vi "Dashboard Main.vi"() -> ()   [LabVIEW 2019]
uses:
  <vilib>/Utility/miscctls.llb/LVRowAndColumnTypeDef.ctl
  <vilib>/event_ctls.llb/eventvkey.ctl
  <vilib>/MakerHub/LINX/Public/Peripherals/Analog/Analog Read 1 Chan.vi
  <vilib>/MakerHub/LINX/Public/Peripherals/Analog/Analog Read N Chans.vi
  <vilib>/MakerHub/LINX/Private/Local IO/LinxAnalogRead.vi
  <vilib>/MakerHub/LINX/Public/Utilities/Check Channel.vi
  <vilib>/Rock Robotics/Network Tables/NT Read Numeric Array.vi
  <vilib>/Rock Robotics/WPI/Dashboard/WPI_DashboardLogging Global.vi
  <vilib>/MakerHub/LINX/Public/Utilities/Open Serial.vi
  <vilib>/MakerHub/LINX/Private/Utilties/Generate Error.vi
  <vilib>/MakerHub/LINX/LMH-LINX.lvlib
panel:
  in  "Camera Settings Right":T1={"Frame Rate"=30, "Compression"=30, "Size"=1, "DB Camera Config"=FALSE} {"Frame Rate" scale=1.0..30.0; "Compression" scale=100.0..-1.0; "Size" items=["640x480", "320x240", "160x120"]}
  in  "Camera Name Right":string(combo)="No Camera Selection"
  out "Camera Perf":string
  in  "Camera Settings":T1={"Frame Rate"=30, "Compression"=30, "Size"=1, "DB Camera Config"=FALSE} {"Frame Rate" scale=1.0..30.0; "Compression" scale=100.0..-1.0; "Size" items=["640x480", "320x240", "160x120"]}
  in  "TCP":refnum<k5>
  in  "Rec Mode":enum32{"Stop", "Record", "Playback"}(radio)
  out "Robot IP":string
  out "Image Message":string="Timeout in Camera Communications"
  in  "Dashboard Tab":T2(tab)
  in  "Select Auto":string(combo)="Select Autonomous ..."
  out "NT Connection":bool
  out "MotorChart R":cluster{"Numeric":dbl, "Numeric":dbl}(graph)
  out "MotorChart L":cluster{"Numeric":dbl, "Numeric":dbl}(graph)
  out "MotorSliders R":cluster{"MotorSlide1":dbl, "MotorSlide2":dbl} {"MotorSlide2" scale=-1.0..1.0 scale format="%#_2e"; "MotorSlide1" scale=-1.0..1.0 scale format="%#_2e"}
  out "MotorSliders L":cluster{"MotorSlide1":dbl, "MotorSlide2":dbl} {"MotorSlide2" scale=-1.0..1.0 scale format="%#_2e"; "MotorSlide1" scale=-1.0..1.0 scale format="%#_2e"}
  out "Gyro":dbl(knob) scale=0.0..360.0
  out "JS1 Z":dbl(slide) scale=-1.0..1.0 scale format="%#_2e"
  out "JS1 Graph":cluster{"X":dbl, "Y":dbl}[](graph)
  out "JS1 Buttons":T3
  out "JS2 Z":dbl(slide) scale=-1.0..1.0 scale format="%#_2e"
  out "JS2 Graph":cluster{"X":dbl, "Y":dbl}[](graph)
  out "JS2 Buttons":T3
  out "Mode":T4(ring)=enum."Auto Disabled"
  out "Right Camera Perf":cluster{"Bandwidth (Mbps)":dbl, "FPS":dbl}
  out "Voltage":dbl(slide) scale=0.0..5.0
  out "Camera Image Right":T5(plugin-control)
  in  "DB/String 9":string
  in  "DB/String 8":string
  in  "DB/String 7":string
  in  "DB/String 6":string
  in  "DB/String 5":string
  in  "DB/String 4":string
  in  "DB/String 3":string
  in  "DB/String 2":string
  in  "DB/String 1":string
  in  "DB/String 0":string
  in  "DB/Slider 0":dbl(slide) scale=0.0..5.0
  in  "DB/Slider 1":dbl(slide) scale=0.0..5.0
  in  "DB/Slider 2":dbl(slide) scale=0.0..5.0
  in  "DB/Slider 3":dbl(slide) scale=0.0..5.0
  out "DB/LED 3":bool
  out "DB/LED 2":bool
  out "DB/LED 1":bool
  out "DB/LED 0":bool
  in  "DB/Button 3":bool
  in  "DB/Button 2":bool
  in  "DB/Button 1":bool
  in  "DB/Button 0":bool caption="New Name"
  in  "Test Slider":dbl(slide) scale=0.0..100.0 scale format="%#_3g"
  in  "On/Off":bool caption="Solenoid"
  in  "Test Name":u16(ring) items=["Select the test to run..."]
  in  "Test Tree":string(tree)
  in  "Motor":cluster{"Value":dbl, "Enable":bool} {"Value" scale=-1.0..1.0 scale format="%#_3g"}
  out "Progress":T6 {"Test Progress" scale=0.0..100.0}
  in  "Rev/Fwd":cluster{"Forward":bool, "Reverse":bool}
  in  "Test Ring":u16(ring) items=["Monochrome", "Color"]
  out "Cmd Status":string
  in  "Execute Command":bool
  in  "Command Params":string[][](table)
  in  "Command Selection":i32(listbox)
  in  "CheckList":i32(listbox)
  out "Tree":string(tree)
  out "Camera Image":T5(plugin-control)
  out "Background":bool
  in  "Camera Name":string(combo)="No Camera Selection"
  # "HW"
  # "HW"
  # "Joysticks"
  # "Drive Motors"
  # "Front"
  # "Right"
  # "Left"
  # "Back"
  # "This tab is a great place for autonomous settings and robot-specific values.\nPlace controls and indicators inside this tab and match name to\nDashboard Variables on robot. You can also delete this comment."
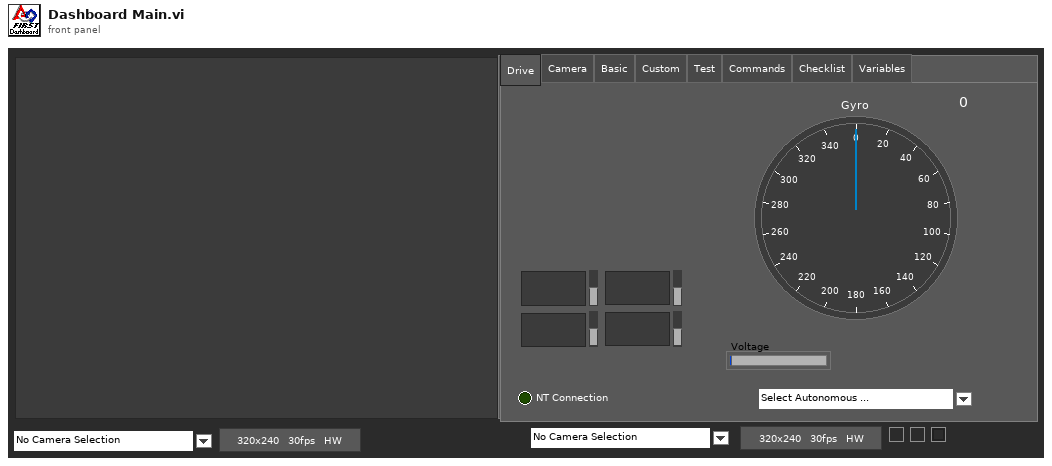
[diagram p1: front panel]
types:
  T1 = cluster{"Frame Rate":i32, "Compression":i32, "Size":u16, "DB Camera Config":bool}
  T2 = enum32{"Drive", "Camera", "Basic", "Custom", "Test", "Commands", "Checklist", "Variables"}
  T3 = cluster{bool, bool, bool, bool, bool, bool, bool, bool, bool, bool, bool, bool}
  T4 = enum8{"Tele-Op Disabled", "Tele-Op Enabled", "Auto Disabled", "Auto Enabled", "Test Disabled", "Test Enabled", "Disconnected", "No Code", "E-Stop"}
  T5 = typedef "IMAQ Image.ctl" = refnum<image>
  T6 = cluster{"Test Progress":u8, "Test Progress Text":string}
  T7 = cluster{"Save Path":path, "Interval (s)":dbl, "Keep":i32}
  T8 = typedef "Image Type" = u32
  T9 = cluster{"IDs":cluster{"RPC field ID":u16, "Unique ID":u16}, "String":string}
  T10 = typedef "LMH-LINX.lvlib/LINX Ref.ctl" = cluster{"IO":T11, "Interface":T12, "LINX Device Config":T13}
  T11 = typedef "LMH-LINX.lvlib/Platform.ctl" = enum16{"Remote", "Local"}
  T12 = typedef "LMH-LINX.lvlib/Interface.ctl" = enum16{"Serial", "TCP"}
  T13 = typedef "LMH-LINX.lvlib/Device.lvlib/LINX Device Config.ctl" = cluster{"Interface":T12, "COM Port":refnum<visa-resource-name>, "TCP Configuration":T14, "Device Family":u8, "Device ID":u8, "Device Name":string, "TCP Ref":refnum<k5>, "Channels":T15}
  T14 = typedef "LMH-LINX.lvlib/Device.lvlib/TCP Config.ctl" = cluster{"IP Address":string, "Port":u16}
  T15 = typedef "LMH-LINX.lvlib/Channels.ctl" = cluster{"DI":u8[], "DO":u8[], "AI":u8[], "AO":u8[], "PWM":u8[], "QE":u8[], "UART":u8[], "I2C 2":u8[], "SPI":u8[], "CAN":u8[], "Servo":u8[], "AI Ref (V)":dbl, "AI Resolution (Bits)":u8, "AO Ref (V)":dbl, "AO Resolution (Bits)":u8}
  T16 = cluster{"Error Strings":string, "Disable Counts":cluster{u16, u16}, "Rail Faults":cluster{u16, u16, u16}, "Robot IP":string, "DB Mode":u8, "Event Info":cluster{"Name":string, "Type":u8, "Number":u16, "Replay":u8}}
  T17 = cluster{"Storage":cluster{"Disk Free":u64, "RAM Block":u32, "RAM free":u32}, "CPU Utilization":cluster{"CPU % ISR":sgl, "CPU % Time Crit":sgl, "CPU % Timed Str":sgl, "CPU % High":sgl, "CPU % Above":sgl, "CPU % Normal":sgl, "CPU % Low":sgl}, "CAN":cluster{"% Bus Utilization":sgl, "Bus Off Cnt":u32, "TX_FIFO Full Cnt":u32, "Receive Error Cnt":u8, "Transmit Error Cnt":u8}, "HID":cluster{"HID Outputs":u32, "Rumble Low":u16, "Rumble High":u16}[]}
  T18 = cluster{"Status bits":cluster{"Test Mode":bool, "Autonomous":bool, "Enabled":bool, "Code Start":bool, "Brownout":bool, "Reserved 2":bool, "Reserved 3":bool, "E-Stop":bool}, "Code Trace":cluster{"Disabled":bool, "TeleOp":bool, "Auto":bool, "Test":bool}, "Controller Type":enum16{"unknown", "cRIO", "roboRio"}, "Code?":enum16{"unknown", "noCode", "code"}, "Battery V":dbl}
  T19 = cluster{"Control Bits":cluster{"TestMode":bool, "Autonomous":bool, "Enabled":bool, "FMS Present":bool, bool, bool, bool, "E-Stop":bool}, "Team Station ":u8, "Countdown":sgl, "Joystick Values":cluster{"Axes":dbl[], "Buttons":bool[], "POVs":i16[]}[]}
  T20 = cluster{"Axes":dbl[], "Buttons":bool[], "POVs":i16[]}[]
  T21 = cluster{"Axes":dbl[], "Buttons":bool[], "POVs":i16[]}
  T22 = cluster{"Buttons[0]":bool, "Buttons[1]":bool, "Buttons[2]":bool, "Buttons[3]":bool, "Buttons[4]":bool, "Buttons[5]":bool, "Buttons[6]":bool, "Buttons[7]":bool, "Buttons[8]":bool, "Buttons[9]":bool, "Buttons[10]":bool, "Buttons[11]":bool}
  T23 = cluster{"Camera Image":refnum<vi>, "Dashboard Tab":refnum<vi>, "Background":refnum<vi>, "Rec Mode":refnum<vi>, "Test Slider":refnum<vi>, "On/Off ":refnum<vi>, "Test Ring":refnum<vi>, "Rev/Fwd":refnum<vi>, "Test Name":refnum<vi>, "Motor":refnum<vi>, "Progress":refnum<vi>, "CheckList":refnum<vi>, "Tree":refnum<vi>, "Test Tree":refnum<vi>, "Command Params":refnum<vi>, "Command Selection":refnum<vi>, "Execute Command":refnum<vi>, "Cmd Status":refnum<vi>, "Camera Settings":refnum<vi>, "Camera Name":refnum<vi>, "Camera Perf":refnum<vi>, "Camera Settings Right":refnum<vi>, "Camera Name Right":refnum<vi>, "Camera Image Right":refnum<vi>}
  T24 = cluster{"Global Rectangle":i32[], "Contours":cluster{"Contour Type":u32, "ROI Type":u32, "Points":i32[]}[]}
  T25 = cluster{"Camera Name":string, string, "Saved DB Images Info":cluster{"Save Path":path, "Interval (s)":dbl, "Keep":i32}}
  T26 = cluster{"Camera Name Right":string, string, "Saved DB Images Info":cluster{"Save Path":path, "Interval (s)":dbl, "Keep":i32}}
  T27 = cluster{"Operation":enum16{"Update", "Clear"}, "Color Box":u32}[]
  T28 = typedef "eventvkey.ctl" = enum16{"ASCII", "Enter", "Return", "Shift", "Ctrl", "Alt", "Cmd", "Opt", "Caps", "NumLock", "Clear", "Break", "Up", "Down", "Left", "Right", "Insert", "Delete", "Home", "End", "PageUp", "PageDown", "Escape", "Help", "Pause", "ScrollLock", "F1", "F2", "F3", "F4", "F5", "F6", "F7", "F8", "F9", "F10", "F11", "F12", "F13", "F14", "F15", "F16", "F17", "F18", "F19", "F20", "F21", "F22", "F23", "F24", "Play", "VolumeUp", "VolumeDown", "Mute", "Two Byte Char"}
  T29 = cluster{"Image Size":bool, "Image Type":bool, "Pixel Value":bool, "ROI Information":bool, "Zoom Factor":bool}
  T30 = cluster{"Operation":enum16{"Update", "Clear"}, "Color Box":u32}
  T31 = typedef "LVRowAndColumnTypeDef.ctl" = cluster{"Row":i32, "Column":i32}
  T32 = cluster{"Shift":bool, "Ctrl":bool, "Alt":bool, "Cmd":bool, "Opt":bool}
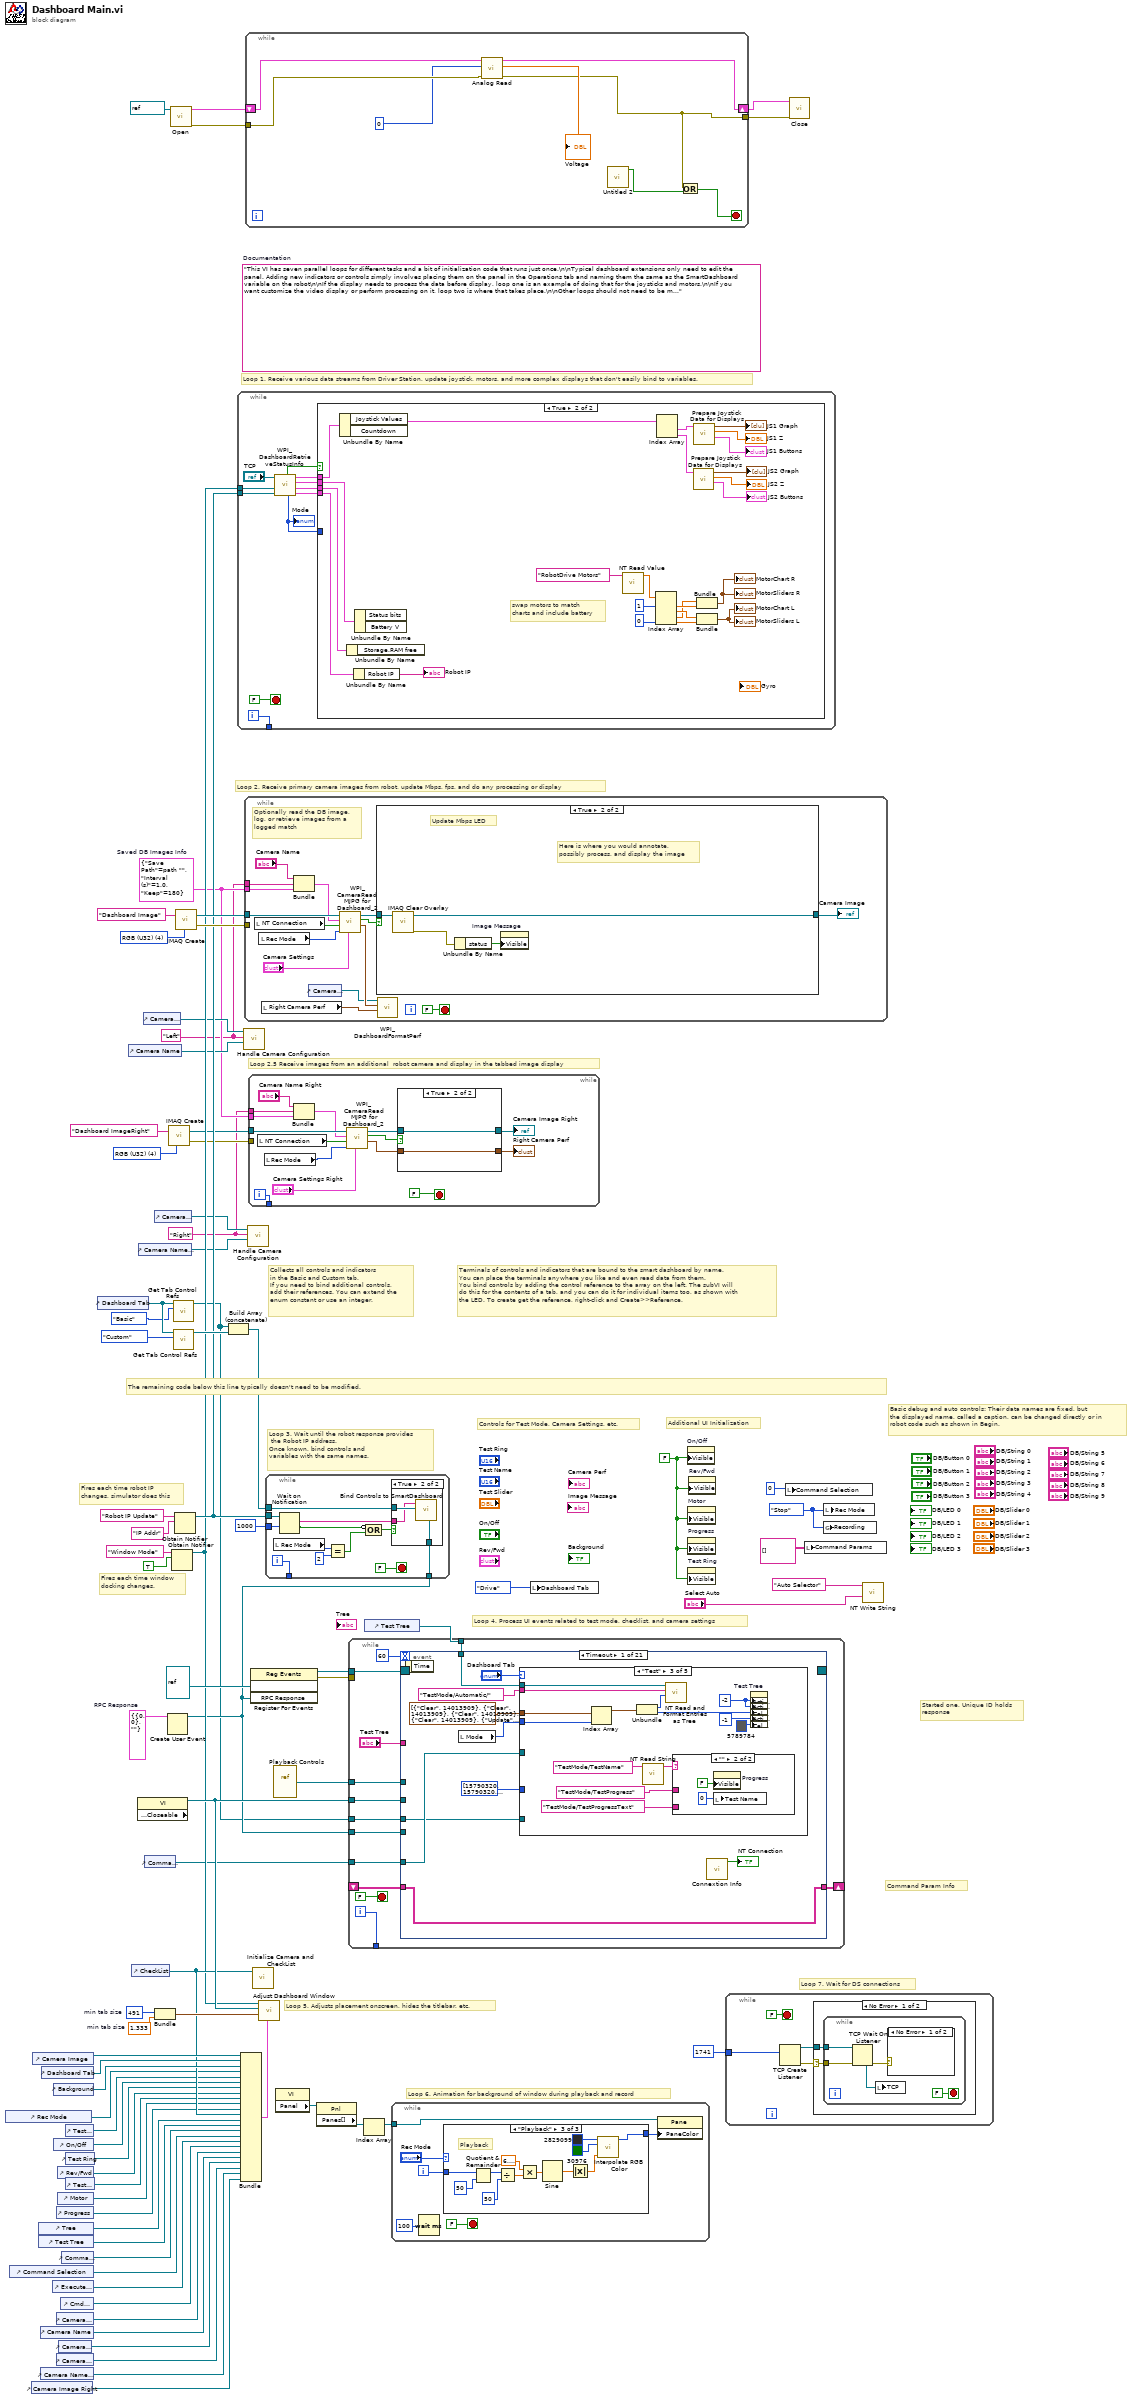
[diagram p0: block diagram]
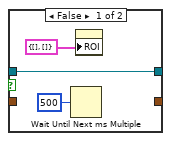
[diagram p2: hidden frame]
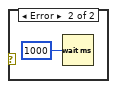
[diagram p3: hidden frame]
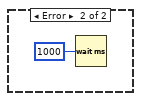
[diagram p4: hidden frame]
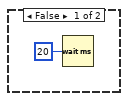
[diagram p5: hidden frame]
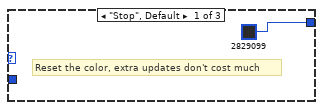
[diagram p6: hidden frame]
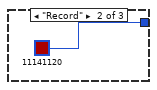
[diagram p7: hidden frame]
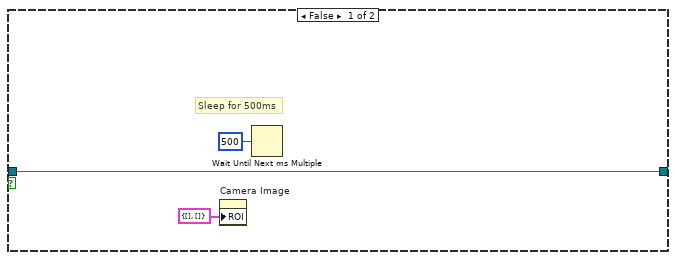
[diagram p9: hidden frame]
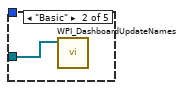
[diagram p11: hidden frame]
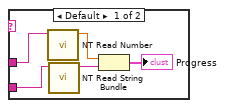
[diagram p12: hidden frame]
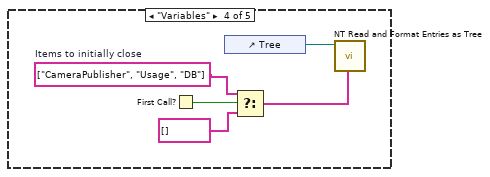
[diagram p13: hidden frame]
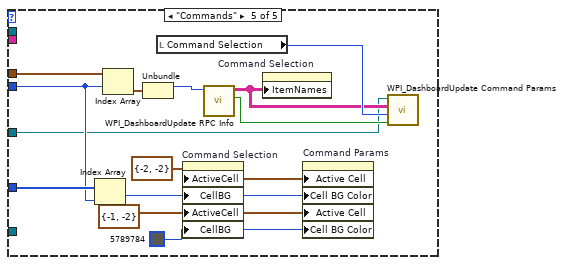
[diagram p14: hidden frame]
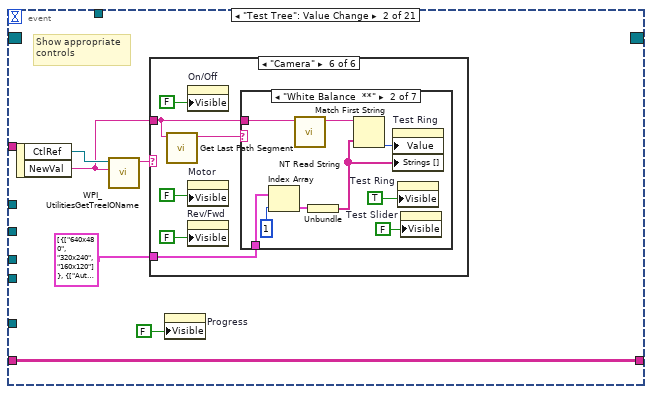
[diagram p15: hidden frame]
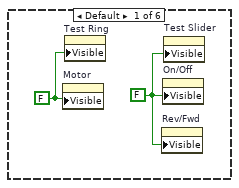
[diagram p16: hidden frame]
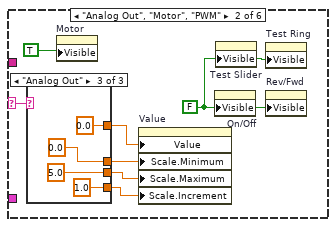
[diagram p17: hidden frame]
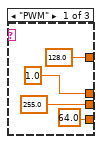
[diagram p18: hidden frame]
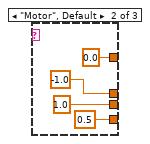
[diagram p19: hidden frame]
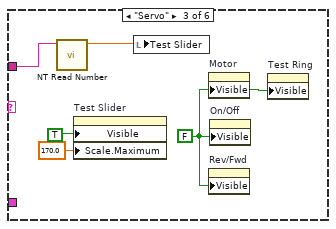
[diagram p20: hidden frame]
diagram:
  w8 = T7 {"Save Path"=path "", "Interval (s)"=1.0, "Keep"=180}  # Saved DB Images Info
  w7 = "Right"
  w6 = "Left"
  w18 = T8 4 items=["Grayscale (U8)", "Grayscale (I16)", "Grayscale (SGL)", "Complex (CSG)", "RGB (U32)", "HSL (U32)", "RGB (U64)"] ("Image Type")
  w34 = T9 {"IDs"={"RPC field ID"=0, "Unique ID"=0}, "String"=""}  # RPC Response
  w57 = 491  # min tab size
  w56 = 1.333  # min tab size
  w64 = enum32{"Stop", "Record", "Playback"}."Stop" ("Rec Mode")
  w41 = FALSE ("Visible")
  (unwired) "This VI has seven parallel loops for different tasks and a bit of initialization code that runs just once.\n\nTypical dashboard extensions only need to edit the panel. Adding new indicators or controls simply involves placing them on the panel in the Operations tab and naming them the same as the SmartDashboard variable on the robot\n\nIf the display needs to process the data before display, loop one is an example of doing that for the joysticks and motors.\n\nIf you want customize the video display or perform processing on it, loop two is where that takes place.\n\nOther loops should not need to be modified. They are pretty standard, and document the task they perform."  # Documentation
  w81 = T8 4 items=["Grayscale (U8)", "Grayscale (I16)", "Grayscale (SGL)", "Complex (CSG)", "RGB (U32)", "HSL (U32)", "RGB (U64)"] ("Image Type")
  # "Loop 2.5 Receive images from an additional  robot camera and display in the tabbed image display"
  # "Command Param Info"
  # "Started one, Unique ID holds\nresponse"
  # "Loop 7. Wait for DS connections"
  # "Basic debug and auto controls: Their data names are fixed, but\nthe displayed name, called a caption, can be changed directly or in\nrobot code such as shown in Begin."
  # "Controls for Test Mode, Camera Settings, etc."
  # "Additional UI Initialization"
  # "Loop 6. Animation for background of window during playback and record"
  # "Fires each time robot IP\nchanges, simulator does this"
  # "Fires each time window\ndocking changes."
  # "Collects all controls and indicators\nin the Basic and Custom tab.\nIf you need to bind additional controls,\nadd their references. You can extend the\nenum constant or use an integer."
  # "The remaining code below this line typically doesn't need to be modified."
  # "Loop 4. Process UI events related to test mode, checklist, and camera settings"
  # "Terminals of controls and indicators that are bound to the smart dashboard by name.\nYou can place the terminals anywhere you like and even read data from them.\nYou bind controls by adding the control reference to the array on the left. The subVI will\ndo this for the contents of a tab, and you can do it for individual items too, as shown with\nthe LED. To create get the reference, right-click and Create>>Reference."
  # "Loop 3. Wait until the robot response provides\n the Robot IP address.\nOnce known, bind controls and\nvariables with the same names."
  # "Loop 5. Adjusts placement onscreen, hides the titlebar, etc."
  # "Loop 1. Receive various data streams from Driver Station, update joystick, motors, and more complex displays that don't easily bind to variables."
  # "Loop 2. Receive primary camera images from robot, update Mbps, fps, and do any processing or display"
  n1 = control-ref of="Rec Mode"() -> (w47:refnum<vi>)
  n2 = control-ref of="Command Selection"() -> (w33:refnum<vi>)
  n3 = control-ref of="Camera Image Right"() -> (w11:refnum<vi>)
  n4 = control-ref of="Camera Image"() -> (w59:refnum<vi>)
  n5 = control-ref of="Tree"() -> (w51:refnum<vi>)
  n6 = control-ref of="Test Tree"() -> (w50:refnum<vi>)
  n7 = control-ref of="Camera Name"() -> (w24:refnum<vi>)
  n8 = control-ref of="Camera Name Right"() -> (w12:refnum<vi>)
  n9 = control-ref of="Dashboard Tab"() -> (w58:refnum<vi>)
  n10 = control-ref of="Execute Command"() -> (w35:refnum<vi>)
  n11 = control-ref of="Background"() -> (w54:refnum<vi>)
  n12 = control-ref of="On/Off"() -> (w45:refnum<vi>)
  n13 = control-ref of="Progress"() -> (w42:refnum<vi>)
  n14 = control-ref of="Camera Settings"() -> (w25:refnum<vi>)
  n15 = control-ref of="Camera Settings Right"() -> (w13:refnum<vi>)
  n16 = control-ref of="Rev/Fwd"() -> (w43:refnum<vi>)
  n17 = control-ref of="Motor"() -> (w48:refnum<vi>)
  n18 = control-ref of="Camera Perf"() -> (w23:refnum<vi>)
  n19 = control-ref of="Cmd Status"() -> (w29:refnum<vi>)
  n20 = control-ref of="Command Params"() -> (w36:refnum<vi>)
  n21 = control-ref of="Test Slider"() -> (w46:refnum<vi>)
  n22 = control-ref of="Test Ring"() -> (w44:refnum<vi>)
  n23 = control-ref of="Test Name"() -> (w49:refnum<vi>)
  n24 = control-ref of="Dashboard Tab"() -> (w62:refnum<vi>)
  n25 = control-ref of="Camera Name"() -> (w26:refnum<vi>)
  n26 = control-ref of="CheckList"() -> (w52:refnum<vi>)
  n27 = property class="VI" props=["Front Panel.Closeable"]() -> (reference out=w63:refnum<vi>)  [unwired: 2 in, 2 out]
  n28 = control-ref of="Camera Name Right"() -> (w14:refnum<vi>)
  n29 = control-ref of="Camera Settings"() -> (w27:refnum<vi>)
  n30 = control-ref of="Command Params"() -> (w28:refnum<vi>)
  n31 = control-ref of="Camera Settings Right"() -> (w15:refnum<vi>)
  n32 = Bundle("min tab size"=w57, "min tab size"=w56) -> (w55:cluster{"min tab size":i32, "min tab size":dbl})  [unwired: 1 in]
  n33 = Create User Event(user event datatype=w34) -> (user event=w30:refnum<user-event>)  [unwired: 1 in, 1 out]
  n34 = call "IMAQ Create"("Image Name"="Dashboard ImageRight", "Image Type"=w18) -> ("New Image"=w17:T5, "error out"=w16:errorcluster)  [unwired: 2 in, 1 out]
  n35 = call-poly <vilib>:"Open.vi"("Serial Port"=refnum<visa-resource-name> "N/A") -> ("Error Out"=w3:errorcluster, "LINX Resource"=w4:T10)  [unwired: 8 in, 1 out]
  n36 = Obtain Notifier(name (unnamed)="Window Mode", notification data type=TRUE) -> (notifier out=w39:refnum<notifier>)  [unwired: 2 in, 2 out]
  n37 = call <vilib>:"Get Tab Control Refs.vi"("Page Index"=T2."Basic" ("Dashboard Tab"), "TabControl in"=w62) -> ("ControlsOnPage"=w22:refnum<vi>[])  [unwired: 9 in]
  n38 = call <vilib>:"Get Tab Control Refs.vi"("Page Index"=T2."Custom" ("Dashboard Tab"), "TabControl in"=w62) -> ("ControlsOnPage"=w61:refnum<vi>[])  [unwired: 9 in]
  n39 = Obtain Notifier(name (unnamed)="Robot IP Update", notification data type="IP Addr" ("name (unnamed)")) -> (notifier out=w40:refnum<notifier>)  [unwired: 2 in, 2 out]
  n40 = call "IMAQ Create"("Image Name"="Dashboard Image", "Image Type"=w81) -> ("New Image"=w79:T5, "error out"=w78:errorcluster)  [unwired: 2 in, 1 out]
  n41 = Build Array (concatenate)(w22, w61) -> (w60:refnum<vi>[])
  n42 = while {
    tunnel: [w91] -> _
    tunnel: w40 -> [w85]
    tunnel: w39 -> [w82]
    i -> [w91]
    stop <- FALSE stop-if-true
    n43 = call <vilib>:"WPI_DashboardRetrieveStatusInfo.vi"("Binding Refnum"=w85, "Window Mode Notifier"=w82, "TCP Cnx"="TCP") -> ("Power and Errors"=w86:T16, "Robot Metrics"=w89:T17, "Status Info"=w90:T18, "Control Info"=w87:T19, "Robot Mode"=w84:T4, "Process?"=w88:bool)  [unwired: 3 in]
    "Mode" <- w84
    n44 = case shown="True" w88 {
      tunnel: w90 -> [_ w117]
      tunnel: w89 -> [_ w116]
      tunnel: w87 -> [_ w115]
      tunnel: w86 -> [_ w114]
      tunnel: w84 -> [_ _]
      frame False {
        n45 = Wait (ms)(milliseconds to wait=u32 20) -> ()  [unwired: 1 out]
      }
      frame True {
        # "swap motors to match\ncharts and include battery"
        n46 = Unbundle By Name(w115) -> ("Joystick Values"=w105:T20)  [unwired: 1 out]
        n47 = Unbundle By Name(w116) -> ()  [unwired: 1 out]
        n48 = Unbundle By Name(w114) -> ("Robot IP"=→"Robot IP":string)
        n49 = Unbundle By Name(w117) -> ()  [unwired: 2 out]
        n50 = call-poly <vilib>:"NT Read Value.vi"("Name"="RobotDrive Motors") -> ("Numeric Array"=w95:dbl[])  [unwired: 9 in, 1 out]
        n51 = Index Array(array=w95, index #1=1, index #4=0) -> (element #1=w109:dbl, element #2=w110:dbl, element #3=w108:dbl, element #4=w113:dbl)  [unwired: 2 in]
        n52 = Index Array(array=w105) -> (element #1=w104:T21, element #2=w100:T21)  [unwired: 2 in]
        n53 = call "Prepare Joystick Data for Displays.vi"("Joystick Values"=w100) -> ("Buttons"=→"JS2 Buttons":T22, "Z Axis"=→"JS2 Z":dbl, "Cartesian Data"=→"JS2 Graph":cluster{"X axis":dbl, "X axis":dbl}[])  [unwired: 8 in]
        n54 = call "Prepare Joystick Data for Displays.vi"("Joystick Values"=w104) -> ("Buttons"=→"JS1 Buttons":T22, "Z Axis"=→"JS1 Z":dbl, "Cartesian Data"=→"JS1 Graph":cluster{"X axis":dbl, "X axis":dbl}[])  [unwired: 8 in]
        n55 = Bundle("Numeric"=w108, "Numeric"=w109) -> (→"MotorChart R" →"MotorSliders R":cluster{"Numeric":dbl, "Numeric":dbl})  [unwired: 1 in]
        n56 = Bundle("Numeric"=w110, "Numeric"=w113) -> (→"MotorChart L" →"MotorSliders L":cluster{"Numeric":dbl, "Numeric":dbl})  [unwired: 1 in]
      }
    }
  }
  n57 = Bundle("Camera Image"=w59, "Dashboard Tab"=w58, "Background"=w54, "Rec Mode"=w47, "Test Slider"=w46, "On/Off"=w45, "Test Ring"=w44, "Rev/Fwd"=w43, "Test Name"=w49, "Motor"=w48, "Progress"=w42, "CheckList"=w52, "Tree"=w51, "Test Tree"=w50, "Command Params"=w36, "Command Selection"=w33, "Execute Command"=w35, "Cmd Status"=w29, "Camera Settings"=w25, "Camera Name"=w24, "Camera Perf"=w23, "Camera Settings Right"=w13, "Camera Name Right"=w12, "Camera Image Right"=w11) -> (w53:T23)  [unwired: 1 in]
  n58 = call "Handle Camera Configuration.vi"("CameraNameRef"=w26, "Display Name"=w6, "ClusterRef"=w27) -> ()  [unwired: 9 in]
  n59 = while {
    tunnel: w79 -> [w131]
    tunnel: w78 -> [_]
    tunnel: w8 -> [w124]
    tunnel: w6 -> [w121]
    stop <- FALSE stop-if-true
    # "Optionally read the DB image,\nlog, or retrieve images from a\nlogged match"
    n60 = local read "NT Connection"() -> (w125:bool)
    n61 = local read "Rec Mode"() -> (w128:enum32{"Stop", "Record", "Playback"})
    n62 = local read "Right Camera Perf"() -> (w119:cluster{"Bandwidth (Mbps)":dbl, "FPS":dbl})
    n63 = Bundle("Camera Name"="Camera Name", w121, "Saved DB Images Info"=w124) -> (w123:T25)  [unwired: 1 in]
    n64 = control-ref of="Camera Perf"() -> (w118:refnum<vi>)
    n65 = call <vilib>:"WPI_CameraRead MJPG for Dashboard_2.vi"("Camera Settings"="Camera Settings", "Rec Mode"=w128, "NT Connection"=w125, "Capture Info"=w123, "Image in"=w131) -> ("perf info"=w120:cluster{"Bandwidth (Mbps)":dbl, "fps":dbl}, "Active"=w129:bool, "Image\\ out"=w130:T5)  [unwired: 4 in]
    n66 = case shown="True" w129 {
      tunnel: w130 -> [w134 w137]
      tunnel: [w134 w136] -> w126
      frame False {
        # "Sleep for 500ms"
        n67 = property on="Camera Image" class="ImageControl"("ROI"=T24 {"Global Rectangle"=[], "Contours"=[]}) -> ()  [unwired: 2 in, 2 out]
        n68 = Wait Until Next ms Multiple(millisecond multiple=u32 500) -> ()  [unwired: 1 out]
      }
      frame True {
        # "Here is where you would annotate,\npossibly process, and display the image"
        # "Update Mbps LED"
        n69 = call "IMAQ Clear Overlay"("Image"=w137) -> ("error out"=w138:errorcluster, "Image Out"=w136:T5)  [unwired: 2 in, 7 out]
        n70 = Unbundle By Name(w138) -> ("status"=w139:bool)
        n71 = property on="Image Message" class="Str"("Visible"=w139) -> ()  [unwired: 2 in, 2 out]
      }
    }
    "Camera Image" <- w126
    n72 = call <vilib>:"WPI_DashboardFormatPerf.vi"("Right Camera Perf"=w119, "Performance"=w120, "String in"=w118) -> ()  [unwired: 9 in]
  }
  n73 = while {
    shift-right: [w145] -> w1
    shift-left: w4 -> [w146]
    tunnel: w3 -> [w147]
    tunnel: [w142] -> w2
    stop <- w141 stop-if-true
    n74 = call-poly <vilib>:"Analog Read.vi"("Error In"=w147, "Analog Channel"=u8 0, "LINX Resource"=w146) -> ("Error Out"=w142:errorcluster, "Voltage"=→"Voltage":dbl, "LINX Resource"=w145:T10)  [unwired: 5 in, 1 out]
    n75 = call "Untitled 2.vi"() -> ("Boolean"=w140:bool)  [unwired: 11 in]
    n76 = Or(x=w142, y=w140) -> (x .or. y?=w141:bool)
  }
  n77 = call "Handle Camera Configuration.vi"("CameraNameRef"=w14, "Display Name"=w7, "ClusterRef"=w15) -> ()  [unwired: 9 in]
  n78 = while {
    tunnel: w17 -> [w162]
    tunnel: w16 -> [_]
    tunnel: [w157] -> _
    tunnel: w8 -> [w153]
    tunnel: w7 -> [w150]
    i -> [w157]
    stop <- FALSE stop-if-true
    n79 = local read "NT Connection"() -> (w154:bool)
    n80 = local read "Rec Mode"() -> (w161:enum32{"Stop", "Record", "Playback"})
    n81 = Bundle("Camera Name Right"="Camera Name Right", w150, "Saved DB Images Info"=w153) -> (w152:T26)  [unwired: 1 in]
    n82 = call <vilib>:"WPI_CameraRead MJPG for Dashboard_2.vi"("Camera Settings"="Camera Settings Right", "Rec Mode"=w161, "NT Connection"=w154, "Capture Info"=w152, "Image in"=w162) -> ("perf info"=w148:cluster{"Bandwidth (Mbps)":dbl, "fps":dbl}, "Active"=w156:bool, "Image\\ out"=w159:T5)  [unwired: 4 in]
    n83 = case shown="True" w156 {
      tunnel: w159 -> [w164 w167]
      tunnel: [w164 w167] -> w155
      tunnel: [_ w166] -> w149
      tunnel: w148 -> [_ w166]
      frame False {
        n84 = Wait Until Next ms Multiple(millisecond multiple=u32 500) -> ()  [unwired: 1 out]
        n85 = property on="Camera Image Right" class="ImageControl"("ROI"=T24 {"Global Rectangle"=[], "Contours"=[]}) -> ()  [unwired: 2 in, 2 out]
      }
      frame True {
      }
    }
    "Camera Image Right" <- w155
    "Right Camera Perf" <- w149
  }
  n86 = register-events(refnum<vi> refnum, w30) -> (reference out=w68:refnum<event-registration>, error out=w67:errorcluster)  [unwired: 2 in]
  n87 = call "Initialize Camera and CheckList.vi"("ListBox in"=w52) -> ()  [unwired: 11 in]
  n88 = call "Adjust Dashboard Window.vi"("Sizing Refnums"=w53, "Size Constraints"=w55, "VI"=w63, "WIn Mode"=w39) -> ()  [unwired: 8 in]
  n89 = while {
    tunnel: w60 -> [w179]
    tunnel: w40 -> [w177]
    tunnel: [w175] -> _
    tunnel: u32 1000 ("milliseconds to wait") -> [w174]
    tunnel: w30 -> [w168]
    i -> [w175]
    stop <- FALSE stop-if-true
    n90 = local read "Rec Mode"() -> (w170:enum32{"Stop", "Record", "Playback"})
    n91 = Wait on Notification(notifier=w177, timeout in ms (-1)=w174) -> (notification=w176:string, timed out?=w172:bool)  [unwired: 2 in, 2 out]
    n92 = Equal?(x=w170, y=u16 2 ("Rec Mode")) -> (x = y?=w171:bool)
    n93 = Compound Arithmetic op=OR(invert w172, w171) -> (w173:bool)
    n94 = case shown="True" w173 {
      tunnel: w179 -> [_ w182]
      tunnel: w176 -> [_ w181]
      tunnel: w168 -> [_ w180]
      frame False {
      }
      frame True {
        n95 = call <vilib>:"Bind Controls to SmartDashboard.vi"("RPC ref"=w180, "Bound Control Refs"=w182, "Server IP Address"=w181) -> ()  [unwired: 9 in]
      }
    }
  }
  n96 = vi-ref "Playback Controls.vi"() -> (w69:refnum<vi>)
  n97 = property class="VI"() -> ("Panel"=w71:refnum<vi>)  [unwired: 2 in, 2 out]
  n98 = property class="Pnl"(reference=w71) -> ("Panes[]"=w72:refnum<vi>[])  [unwired: 1 in, 2 out]
  n99 = Index Array(array=w72) -> (element=w70:refnum<vi>)  [unwired: 1 in]
  n100 = control-ref of="Test Tree"() -> (w73:refnum<vi>)
  n101 = while {
    tunnel: [w192] -> _
    tunnel: w73 -> [w191]
    tunnel: w69 -> [w190]
    tunnel: w68 -> [w189]
    tunnel: w67 -> [_]
    tunnel: w63 -> [w188]
    tunnel: w30 -> [w187]
    tunnel: w28 -> [w186]
    shift-right: [w185] -> _
    shift-left: _ -> [w184]
    tunnel: w22 -> [w183]
    i -> [w192]
    stop <- FALSE stop-if-true
    n102 = event shown="[0] Timeout" {
      selector: w189 -> [_ _ _ _ _ _ _ _ _ _ _ _ _ _ _ _ _ _ _ _ _]
      dyn-events: [_ _ _ _ _ _ _ _ _ _ _ _ _ _ _ _ w452 _ _ _ _] -> _
      timeout: u32 60 ("milliseconds to wait") -> [_ _ _ _ _ _ _ _ _ _ _ _ _ _ _ _ _ _ _ _ _]
      tunnel: w191 -> [w204 _ _ _ _ _ _ _ _ _ _ _ _ _ _ _ _ _ _ _ _]
      tunnel: "Test Tree" -> [_ _ _ _ _ _ _ _ _ _ _ w419 w427 w429 w433 w441 _ _ _ _ _]
      tunnel: w190 -> [_ _ _ _ _ _ _ _ _ _ _ _ _ _ _ _ w454 _ w472 _ _]
      tunnel: w188 -> [_ _ _ _ _ _ _ _ _ _ _ _ _ _ _ _ w450 _ _ _ _]
      tunnel: w187 -> [_ _ _ _ _ _ _ _ _ _ _ _ _ _ _ _ w448 _ _ _ _]
      tunnel: w186 -> [w199 _ _ _ _ _ w370 _ _ _ _ _ _ _ _ _ _ _ _ _ _]
      tunnel: [w198 w247 w349 w354 w363 w367 w368 w377 w387 w394 w406 w418 w425 w428 w432 w440 w447 w467 w469 w473 w486] -> w185
      tunnel: w184 -> [w198 w247 w349 w354 w363 w367 w368 _ _ w394 w406 w418 w425 w428 w432 w440 w447 w467 w469 w473 w486]
      tunnel: w183 -> [w196 _ _ _ _ _ _ _ _ _ _ _ _ _ _ _ _ _ _ _ _]
      event Timeout {
        n103 = event-data() -> ()  [unwired: 1 in, 1 out]
        n104 = local read "Mode"() -> (w201:T4)
        n105 = case shown="\"Test\"" "Dashboard Tab" {
          tunnel: w204 -> [_ _ w220 _ _]
          tunnel: "TestMode/Automatic/" ("Name Pattern") -> [_ _ w219 _ _]
          tunnel: T27 [{"Operation"=enum."Clear", "Color Box"=14013909}, {"Operation"=enum."Clear", "Color Box"=14013909}, {"Operation"=enum."Clear", "Color Box"=14013909}, {"Operation"=enum."Clear", "Color Box"=14013909}, {"Operation"=enum."Update", "Color Box"=14013909}, {"Operation"=enum."Update", "Color Box"=16777215}, {"Operation"=enum."Clear", "Color Box"=14013909}, {"Operation"=enum."Clear", "Color Box"=14013909}, {"Operation"=enum."Clear", "Color Box"=14013909}] -> [_ _ w212 _ w240]
          tunnel: w201 -> [_ _ w211 _ w239]
          tunnel: u32[] [15790320, 15790320, 15790320, 15790320, 16777215, 16777215, 15790320, 15790320, 15790320] -> [_ _ _ _ w245]
          tunnel: w199 -> [_ _ _ _ w233]
          tunnel: w196 -> [_ w206 _ _ _]
          frame "Custom", Default {
          }
          frame "Basic" {
            n106 = call <vilib>:"WPI_DashboardUpdateNames.vi"("Controls on Tab"=w206) -> ()  [unwired: 11 in]
          }
          frame "Test" {
            w218 = -2 ("Active Item:Row Number")
            n107 = Index Array(array=w212, index=w211) -> (element=w213:T30)
            n108 = Unbundle(w213) -> ("Operation"=w214:enum16{"Update", "Clear"}, "Color Box"=w215:u32)
            n109 = call <vilib>:"NT Read String.vi"("Name"="TestMode/TestName") -> ("String"=w209:string)  [unwired: 9 in, 1 out]
            n110 = call <vilib>:"NT Read and Format Entries as Tree.vi"("Operation"=w214, "Name Pattern"=w219, "Tree Refnum"=w220) -> ()  [unwired: 7 in, 2 out]
            n111 = case shown="\"\"" w209 {
              tunnel: "TestMode/TestProgress" ("Name") -> [w222 _]
              tunnel: "TestMode/TestProgressText" ("Name") -> [w221 _]
              frame Default {
                n112 = call <vilib>:"NT Read Number.vi"("Name"=w222) -> ("Numeric"=w223:dbl)  [unwired: 9 in, 1 out]
                n113 = call <vilib>:"NT Read String.vi"("Name"=w221) -> ("String"=w224:string)  [unwired: 9 in, 1 out]
                n114 = Bundle("Numeric"=w223, "String"=w224) -> (→"Progress":cluster{"Numeric":dbl, "String":string})  [unwired: 1 in]
              }
              frame "" {
                n115 = property on="Progress" class="Clust (strict)"("Visible"=FALSE) -> ()  [unwired: 2 in, 2 out]
                n116 = local write "Test Name"(u16 0) -> ()
              }
            }
            n117 = property on="Test Tree" class="Tree (strict)"("Active Item Row Number"=w218, "ActiveColNum"=w218, "CellBG"=w215, "Active Item Row Number"=-1 ("Active Item:Row Number"), "CellBG"=u32 5789784 ("Color Box")) -> ()  [unwired: 2 in, 2 out]
          }
          frame "Variables" {
            w230 = string[] ["CameraPublisher", "Usage", "DB"]  # Items to initially close
            n118 = First Call?() -> (First Call?: T/F=w231:bool)
            n119 = control-ref of="Tree"() -> (w232:refnum<vi>)
            n120 = Select(t=w230, s=w231, f=string[] []) -> (s? t:f=w228:string[])
            n121 = call <vilib>:"NT Read and Format Entries as Tree.vi"("Tags to  Close"=w228, "Tree Refnum"=w232) -> ()  [unwired: 8 in, 2 out]
          }
          frame "Commands" {
            w241 = u32 5789784 ("Color Box")
            w242 = T31 {"Row"=-1, "Column"=-2} ("Active Cell:Active Cell")
            w244 = T31 {"Row"=-2, "Column"=-2} ("Active Cell:Active Cell")
            n122 = Index Array(array=w245, index=w239) -> (element=w243:u32)
            n123 = Index Array(array=w240, index=w239) -> (element=w238:T30)
            n124 = Unbundle(w238) -> ("Operation"=w237:enum16{"Update", "Clear"})  [unwired: 1 out]
            n125 = local read "Command Selection"() -> (w236:i32)
            n126 = property on="Command Selection" class="MCListbox (strict)"("ActiveCell"=w244, "CellBG"=w243, "ActiveCell"=w242, "CellBG"=w241) -> ()  [unwired: 2 in, 2 out]
            n127 = call <vilib>:"WPI_DashboardUpdate RPC Info.vi"("Operation"=w237) -> ("update"=w235:bool, "commands"=w234:string[][])  [unwired: 9 in]
            n128 = property on="Command Selection" class="MCListbox (strict)"("ItemNames"=w234) -> ()  [unwired: 2 in, 2 out]
            n129 = property on="Command Params" class="Tbl (strict)"("Active Cell"=w244, "Cell BG Color"=w243, "Active Cell"=w242, "Cell BG Color"=w241) -> ()  [unwired: 2 in, 2 out]
            n130 = call <vilib>:"WPI_DashboardUpdate Command Params.vi"("Update"=w235, "NewVal"=w236, "Commands"=w234, "Param Tbl"=w233) -> ()  [unwired: 7 in, 1 out]
          }
        }
        n131 = call <vilib>:"Connextion Info.vi"() -> ("Connected"=→"NT Connection":bool)  [unwired: 10 in, 1 out]
      }
      event "Test Tree": Value Change {
        # "Show appropriate\ncontrols"
        n132 = event-data() -> ("CtlRef"=w250:refnum<vi>, "NewVal"=w248:string)  [unwired: 1 in]
        n133 = call <vilib>:"WPI_UtilitiesGetTreeIOName.vi"("NewVal"=w248, "TreeControl in"=w250) -> ("I/O Name"=w251:string)  [unwired: 9 in]
        n134 = case shown="\"Camera\"" w251 {
          selector: w251 -> [_ w258 _ w280 w289 _]
          tunnel: w248 -> [_ _ w277 w279 _ w296]
          tunnel: cluster{string[]}[] [{["640x480", "320x240", "160x120"]}, {["Auto", "Fixed indoor", "Fixed outdoor 1", "Fixed outdoor 2", "Fixed fluorescent 1", "Fixed fluorescent 2", "Hold current"]}, {["Auto", "Flicker-free 50 Hz", "Flicker-free 60 Hz", "Hold current"]}, {["None", "Prioritize frame rate", "Prioritize image quality"]}, {["Monochrome", "Color"]}] -> [_ _ _ _ _ w295]
          frame Default {
            w253 = FALSE ("Visible")
            w252 = FALSE ("Visible")
            n135 = property on="Motor" class="Clust (strict)"("Visible"=w252) -> ()  [unwired: 2 in, 2 out]
            n136 = property on="Test Ring" class="Ring (strict)"("Visible"=w252) -> ()  [unwired: 2 in, 2 out]
            n137 = property on="Rev/Fwd" class="Clust (strict)"("Visible"=w253) -> ()  [unwired: 2 in, 2 out]
            n138 = property on="On/Off" class="Bool (strict)"("Visible"=w253) -> ()  [unwired: 2 in, 2 out]
            n139 = property on="Test Slider" class="Slide (strict)"("Visible"=w253) -> ()  [unwired: 2 in, 2 out]
          }
          frame "Analog Out", "Motor", "PWM" {
            w259 = FALSE ("Visible")
            n140 = case shown="\"Analog Out\"" w258 {
              tunnel: [1.0 ("Value") -1.0 ("Value") 0.0 ("Value")] -> w257
              tunnel: [255.0 ("Value") 1.0 ("Value") 5.0 ("Value")] -> w256
              tunnel: [128.0 ("Value") 0.0 ("Value") 0.0 ("Value")] -> w255
              tunnel: [64.0 ("Value") 0.5 ("Value") 1.0 ("Value")] -> w254
              frame "PWM" {
              }
              frame "Motor", Default {
              }
              frame "Analog Out" {
              }
            }
            n141 = property on="Motor" class="Clust (strict)"("Visible"=TRUE) -> ()  [unwired: 2 in, 2 out]
            n142 = property on="Value" class="Slide (strict)"("Value"=w255, "Scale.Minimum"=w257, "Scale.Maximum"=w256, "Scale.Increment"=w254) -> ()  [unwired: 2 in, 2 out]
            n143 = property on="On/Off" class="Bool (strict)"("Visible"=w259) -> ()  [unwired: 2 in, 2 out]
            n144 = property on="Test Slider" class="Slide (strict)"("Visible"=w259) -> ()  [unwired: 2 in, 2 out]
            n145 = property on="Test Ring" class="Ring (strict)"("Visible"=w259) -> ()  [unwired: 2 in, 2 out]
            n146 = property on="Rev/Fwd" class="Clust (strict)"("Visible"=w259) -> ()  [unwired: 2 in, 2 out]
          }
          frame "Servo" {
            w275 = FALSE ("Visible")
            n147 = call <vilib>:"NT Read Number.vi"("Name"=w277) -> ("Numeric"=w276:dbl)  [unwired: 9 in, 1 out]
            n148 = property on="Test Slider" class="Slide (strict)"("Visible"=TRUE, "Scale.Maximum"=170.0 ("Scale.Range:Maximum")) -> ()  [unwired: 2 in, 2 out]
            n149 = local write "Test Slider"(w276) -> ()
            n150 = property on="Motor" class="Clust (strict)"("Visible"=w275) -> ()  [unwired: 2 in, 2 out]
            n151 = property on="Rev/Fwd" class="Clust (strict)"("Visible"=w275) -> ()  [unwired: 2 in, 2 out]
            n152 = property on="On/Off" class="Bool (strict)"("Visible"=w275) -> ()  [unwired: 2 in, 2 out]
            n153 = property on="Test Ring" class="Ring (strict)"("Visible"=w275) -> ()  [unwired: 2 in, 2 out]
          }
          frame "Relay", "Solenoid" {
            w278 = FALSE ("Visible")
            n154 = property on="Motor" class="Clust (strict)"("Visible"=w278) -> ()  [unwired: 2 in, 2 out]
            n155 = property on="Test Slider" class="Slide (strict)"("Visible"=w278) -> ()  [unwired: 2 in, 2 out]
            n156 = Search and Replace String(input string=w279, search string="/Value  **", replace string="/Direction") -> (result string=w285:string)  [unwired: 5 in, 3 out]
            n157 = property on="Test Ring" class="Ring (strict)"("Visible"=w278) -> ()  [unwired: 2 in, 2 out]
            n158 = call <vilib>:"NT Read String.vi"("Name"=w285) -> ("String"=w283:string)  [unwired: 9 in, 1 out]
            n159 = Equal?(x="Both directions", y=w283) -> (x = y?=w281:bool)
            n160 = Not(x=w281) -> (.not. x?=w282:bool)
            n161 = property on="Rev/Fwd" class="Clust (strict)"("Visible"=w281) -> ()  [unwired: 2 in, 2 out]
            n162 = property on="On/Off" class="Bool (strict)"("Visible"=w282, "Caption.Text"=w280) -> ()  [unwired: 2 in, 2 out]
          }
          frame "Compressor", "Digital Out" {
            w288 = FALSE ("Visible")
            # "Get direction and finish"
            n163 = property on="Motor" class="Clust (strict)"("Visible"=w288) -> ()  [unwired: 2 in, 2 out]
            n164 = property on="Test Slider" class="Slide (strict)"("Visible"=w288) -> ()  [unwired: 2 in, 2 out]
            n165 = property on="Test Ring" class="Ring (strict)"("Visible"=w288) -> ()  [unwired: 2 in, 2 out]
            n166 = property on="On/Off" class="Bool (strict)"("Visible"=TRUE, "Caption.Text"=w289) -> ()  [unwired: 2 in, 2 out]
            n167 = property on="Rev/Fwd" class="Clust (strict)"("Visible"=FALSE) -> ()  [unwired: 2 in, 2 out]
          }
          frame "Camera" {
            n168 = call <vilib>:"Get Last Path Segment.vi"("String in"=w296) -> ("String out"=w297:string)  [unwired: 10 in]
            n169 = property on="On/Off" class="Bool (strict)"("Visible"=FALSE) -> ()  [unwired: 2 in, 2 out]
            n170 = property on="Motor" class="Clust (strict)"("Visible"=FALSE) -> ()  [unwired: 2 in, 2 out]
            n171 = property on="Rev/Fwd" class="Clust (strict)"("Visible"=FALSE) -> ()  [unwired: 2 in, 2 out]
            n172 = case shown="\"White Balance  **\"" w297 {
              tunnel: w296 -> [w303 w312 w321 w330 w339 _ w345]
              tunnel: w295 -> [w301 w309 w318 w327 w336 _ _]
              frame "Size  **" {
                n173 = Index Array(array=w301) -> (element=w300:cluster{string[]})  [unwired: 1 in]
                n174 = call <vilib>:"NT Read String.vi"("Name"=w303) -> ("String"=w302:string)  [unwired: 9 in, 1 out]
                n175 = Unbundle(w300) -> (w298:string[])
                n176 = Match First String(2:w298, 3:w302) -> (0:w299:i32)  [unwired: 1 out]
                n177 = property on="Test Ring" class="Ring (strict)"("Value"=w299, "Strings []"=w298) -> ()  [unwired: 2 in, 2 out]
                n178 = property on="Test Ring" class="Ring (strict)"("Visible"=TRUE) -> ()  [unwired: 2 in, 2 out]
                n179 = property on="Test Slider" class="Slide (strict)"("Visible"=FALSE) -> ()  [unwired: 2 in, 2 out]
              }
              frame "White Balance  **" {
                n180 = Index Array(array=w309, index=1) -> (element=w310:cluster{string[]})
                n181 = call <vilib>:"NT Read String.vi"("Name"=w312) -> ("String"=w311:string)  [unwired: 9 in, 1 out]
                n182 = Unbundle(w310) -> (w307:string[])
                n183 = Match First String(2:w307, 3:w311) -> (0:w306:i32)  [unwired: 1 out]
                n184 = property on="Test Ring" class="Ring (strict)"("Value"=w306, "Strings []"=w307) -> ()  [unwired: 2 in, 2 out]
                n185 = property on="Test Ring" class="Ring (strict)"("Visible"=TRUE) -> ()  [unwired: 2 in, 2 out]
                n186 = property on="Test Slider" class="Slide (strict)"("Visible"=FALSE) -> ()  [unwired: 2 in, 2 out]
              }
              frame "Exposure  **" {
                n187 = Index Array(array=w318, index=2) -> (element=w319:cluster{string[]})
                n188 = call <vilib>:"NT Read String.vi"("Name"=w321) -> ("String"=w320:string)  [unwired: 9 in, 1 out]
                n189 = Unbundle(w319) -> (w315:string[])
                n190 = Match First String(2:w315, 3:w320) -> (0:w316:i32)  [unwired: 1 out]
                n191 = property on="Test Ring" class="Ring (strict)"("Value"=w316, "Strings []"=w315) -> ()  [unwired: 2 in, 2 out]
                n192 = property on="Test Ring" class="Ring (strict)"("Visible"=TRUE) -> ()  [unwired: 2 in, 2 out]
                n193 = property on="Test Slider" class="Slide (strict)"("Visible"=FALSE) -> ()  [unwired: 2 in, 2 out]
              }
              frame "Exposure Priority  **" {
                n194 = Index Array(array=w327, index=3) -> (element=w328:cluster{string[]})
                n195 = call <vilib>:"NT Read String.vi"("Name"=w330) -> ("String"=w329:string)  [unwired: 9 in, 1 out]
                n196 = Unbundle(w328) -> (w324:string[])
                n197 = Match First String(2:w324, 3:w329) -> (0:w325:i32)  [unwired: 1 out]
                n198 = property on="Test Ring" class="Ring (strict)"("Value"=w325, "Strings []"=w324) -> ()  [unwired: 2 in, 2 out]
                n199 = property on="Test Ring" class="Ring (strict)"("Visible"=TRUE) -> ()  [unwired: 2 in, 2 out]
                n200 = property on="Test Slider" class="Slide (strict)"("Visible"=FALSE) -> ()  [unwired: 2 in, 2 out]
              }
              frame "Color Enable  **" {
                n201 = Index Array(array=w336, index=4) -> (element=w337:cluster{string[]})
                n202 = call <vilib>:"NT Read String.vi"("Name"=w339) -> ("String"=w338:string)  [unwired: 9 in, 1 out]
                n203 = Unbundle(w337) -> (w333:string[])
                n204 = Match First String(2:w333, 3:w338) -> (0:w334:i32)  [unwired: 1 out]
                n205 = property on="Test Ring" class="Ring (strict)"("Value"=w334, "Strings []"=w333) -> ()  [unwired: 2 in, 2 out]
                n206 = property on="Test Ring" class="Ring (strict)"("Visible"=TRUE) -> ()  [unwired: 2 in, 2 out]
                n207 = property on="Test Slider" class="Slide (strict)"("Visible"=FALSE) -> ()  [unwired: 2 in, 2 out]
              }
              frame Default {
                n208 = property on="Test Ring" class="Ring (strict)"("Visible"=FALSE) -> ()  [unwired: 2 in, 2 out]
                n209 = property on="Test Slider" class="Slide (strict)"("Visible"=FALSE) -> ()  [unwired: 2 in, 2 out]
              }
              frame "Brightness  **", "Color Level  **", "Compression  **", "FPS  **", "Sharpness  **" {
                n210 = call <vilib>:"NT Read Number.vi"("Name"=w345) -> ("Numeric"=w344:dbl)  [unwired: 9 in, 1 out]
                n211 = local write "Test Slider"(w344) -> ()
                n212 = property on="Test Slider" class="Slide (strict)"("Visible"=TRUE, "Scale.Maximum"=100.0 ("Scale.Range:Maximum")) -> ()  [unwired: 2 in, 2 out]
                n213 = property on="Test Ring" class="Ring (strict)"("Visible"=FALSE) -> ()  [unwired: 2 in, 2 out]
              }
            }
          }
        }
        n214 = property on="Progress" class="Clust (strict)"("Visible"=FALSE) -> ()  [unwired: 2 in, 2 out]
      }
      event "Test Name": Mouse Enter {
        # "Populate the ring with the list of tests"
        n215 = event-data() -> ()  [unwired: 1 in, 1 out]
        n216 = call <vilib>:"NT Read String Array.vi"("Name"="TestMode/TestList") -> ("String Array"=w353:string[])  [unwired: 9 in, 1 out]
        n217 = Build Array (concatenate)("Select the test to run...", w353) -> (w352:string[])
        n218 = property on="Test Name" class="Ring (strict)"("Strings []"=w352) -> ()  [unwired: 2 in, 2 out]
      }
      event "Test Name": Value Change {
        w355 = FALSE ("Visible")
        # "Tell the robot the test name to run"
        n219 = event-data() -> ("NewVal"=w359:u16)  [unwired: 1 in]
        n220 = property on="Test Name" class="Ring (strict)"() -> ("Strings []"=w360:string[])  [unwired: 2 in, 2 out]
        n221 = local write "Progress"(T6 {"Test Progress"=0, "Test Progress Text"=""} ("Progress")) -> ()
        n222 = Index Array(array=w360, index=w359) -> (element=w358:string)
        n223 = call <vilib>:"NT Write String.vi"("String"=w358, "Name"="TestMode/TestName") -> ()  [unwired: 9 in, 1 out]
        n224 = property on="Progress" class="Clust (strict)"("Visible"=TRUE) -> ()  [unwired: 2 in, 2 out]
        n225 = property on="Motor" class="Clust (strict)"("Visible"=w355) -> ()  [unwired: 2 in, 2 out]
        n226 = property on="Test Slider" class="Slide (strict)"("Visible"=w355) -> ()  [unwired: 2 in, 2 out]
        n227 = property on="On/Off" class="Bool (strict)"("Visible"=w355) -> ()  [unwired: 2 in, 2 out]
        n228 = property on="Rev/Fwd" class="Clust (strict)"("Visible"=w355) -> ()  [unwired: 2 in, 2 out]
        n229 = property on="Test Ring" class="Ring (strict)"("Visible"=w355) -> ()  [unwired: 2 in, 2 out]
      }
      event "Select Auto": Mouse Enter {
        # "Populate the combo box with the list of autonomous options"
        n230 = event-data() -> ()  [unwired: 1 in, 1 out]
        n231 = call <vilib>:"NT Read String Array.vi"("Name"="Auto List") -> ("String Array"=w362:string[])  [unwired: 9 in, 1 out]
        n232 = property on="Select Auto" class="CmbBox"("Strings[]"=w362) -> ()  [unwired: 2 in, 2 out]
      }
      event "Select Auto": Value Change {
        # "User modified the Auto Selection. Write to NT variable so robot knows."
        n233 = event-data() -> ("NewVal"=w365:string)  [unwired: 1 in]
        n234 = call <vilib>:"NT Write String.vi"("String"=w365, "Name"="Auto Selector") -> ()  [unwired: 9 in, 1 out]
      }
      event "Command Selection": Value Change {
        # "Get the params and show in table"
        n235 = event-data() -> ("NewVal"=w371:i32)  [unwired: 1 in]
        n236 = property on="Command Selection" class="MCListbox (strict)"() -> ("ItemNames"=w369:string[][])  [unwired: 2 in, 2 out]
        n237 = call <vilib>:"WPI_DashboardUpdate Command Params.vi"("NewVal"=w371, "Commands"=w369, "Param Tbl"=w370) -> ()  [unwired: 8 in, 1 out]
      }
      event "Execute Command": Value Change {
        # "Started one, Unique ID holds\nresponse"
        n238 = event-data() -> ()  [unwired: 1 in, 1 out]
        n239 = property on="Command Selection" class="MCListbox (strict)"() -> ("ItemNames"=w382:string[][])  [unwired: 2 in, 2 out]
        n240 = Index Array(array=w382, index (row)="Command Selection", index (col)=0) -> (element=w380:string)
        n241 = call <vilib>:"Invoke Commands.vi"("Command Params"="Command Params", "Function Name"=w380) -> ("Params"=w376:u8, "Started"=w375:bool)  [unwired: 7 in, 1 out]
        n242 = Array Subset(array="Command Params", length (row)=w376) -> (w377:string[][])  [unwired: 3 in]
        n243 = Select(t="Executing" ("Cmd Status"), s=w375, f="" ("Cmd Status")) -> (s? t:f=→"Cmd Status":string)
      }
      event "Command Selection": Double Click {
        n244 = event-data() -> ("Row"=w390:i32)  [unwired: 1 in]
        n245 = property on="Command Selection" class="MCListbox (strict)"() -> ("ItemNames"=w393:string[][])  [unwired: 2 in, 2 out]
        n246 = local read "Command Params"() -> (w389:string[][])
        n247 = Index Array(array=w393, index (row)=w390, index (col)=0) -> (element=w391:string)
        n248 = call <vilib>:"Invoke Commands.vi"("Command Params"=w389, "Function Name"=w391) -> ("Params"=w388:u8, "Started"=w383:bool)  [unwired: 7 in, 1 out]
        n249 = Array Subset(array=w389, length (row)=w388) -> (w387:string[][])  [unwired: 3 in]
        n250 = Select(t="Executing" ("Cmd Status"), s=w383, f="" ("Cmd Status")) -> (s? t:f=w384:string)
        n251 = local write "Cmd Status"(w384) -> ()
      }
      event "CheckList": Double Click {
        # "Shift clears all"
        # "Update symbols on the listbox"
        n252 = event-data() -> ("PlatMods.Shift"=w395:bool, "Row"=w397:i32)  [unwired: 1 in]
        n253 = case shown="True" w395 {
          tunnel: w397 -> [w401 _]
          tunnel: 1 -> [w400 _]
          frame False {
            n254 = property on="CheckList" class="LstBox (strict)"() -> ("Item Symbols"=w399:i32[])  [unwired: 2 in, 2 out]
            n255 = Replace Array Subset(array=w399, new element=w400, index=w401) -> (w398:i32[])
            n256 = property on="CheckList" class="LstBox (strict)"("Item Symbols"=w398) -> ()  [unwired: 2 in, 2 out]
          }
          frame True {
            w402 = 0 ("Top Row")
            n257 = property on="CheckList" class="LstBox (strict)"() -> ("Number of Rows"=w404:u32)  [unwired: 2 in, 2 out]
            n258 = Initialize Array(0, w404) -> (w403:i32[])
            n259 = property on="CheckList" class="LstBox (strict)"("Top Row"=w402, "Value"=w402, "Item Symbols"=w403) -> ()  [unwired: 2 in, 2 out]
          }
        }
      }
      event "CheckList": Key Down {
        # "Update symbols on the listbox\nLeft and right keys check and uncheck"
        n260 = event-data() -> ("VKey"=w408:T28)  [unwired: 1 in]
        n261 = case shown="\"Left\", \"Right\"" w408 {
          selector: w408 -> [w413 _]
          tunnel: eventvkey."Left" ("VKey") -> [w411 _]
          frame "Left", "Right" {
            n262 = Equal?(x=w411, y=w413) -> (x = y?=w412:bool)
            n263 = Select(t=0, s=w412, f=1) -> (s? t:f=w414:i32)
            n264 = property on="CheckList" class="LstBox (strict)"() -> ("Item Symbols"=w417:i32[])  [unwired: 2 in, 2 out]
            n265 = Replace Array Subset(array=w417, new element=w414, index="CheckList") -> (w416:i32[])
            n266 = property on="CheckList" class="LstBox (strict)"("Item Symbols"=w416) -> ()  [unwired: 2 in, 2 out]
          }
          frame Default {
          }
        }
      }
      event "Motor.Enable": Value Change {
        # "When the test mode otor enable helper is set, update that\ntree row item's value"
        n267 = event-data() -> ("NewVal"=w423:bool)  [unwired: 1 in]
        n268 = Unbundle("Motor") -> ("Value"=w422:dbl)  [unwired: 1 out]
        n269 = Select(t=w422, s=w423, f=0.0) -> (s? t:f=w420:dbl)
        n270 = call <vilib>:"NT Write Number.vi"("Numeric"=w420, "Name"=w419) -> ()  [unwired: 9 in, 1 out]
      }
      event "Test Slider": Value Change {
        # "When the test mode slider helper is set, update that\ntree row item's value"
        n271 = event-data() -> ("NewVal"=w426:dbl)  [unwired: 1 in]
        n272 = call <vilib>:"NT Write Number.vi"("Numeric"=w426, "Name"=w427) -> ()  [unwired: 9 in, 1 out]
      }
      event "On/Off": Value Change {
        # "When the test mode on/off helper value is set, update that\ntree row item's value"
        n273 = event-data() -> ("NewVal"=w431:bool)  [unwired: 1 in]
        n274 = Boolean To (0,1)(Boolean=w431) -> (0, 1=w430:i16)
        n275 = call <vilib>:"NT Write Number.vi"("Numeric"=w430, "Name"=w429) -> ()  [unwired: 9 in, 1 out]
      }
      event "Rev/Fwd": Value Change {
        # "When the test mode helper value for relays is set, update that\ntree row item's value"
        n276 = event-data() -> ("NewVal.Forward"=w439:bool, "NewVal.Reverse"=w438:bool)  [unwired: 1 in]
        n277 = Boolean To (0,1)(Boolean=w439) -> (0, 1=w435:i16)
        n278 = Boolean To (0,1)(Boolean=w438) -> (0, 1=w437:i16)
        n279 = Negate(x=w437) -> (-x=w436:i16)
        n280 = Add(x=w435, y=w436) -> (x+y=w434:i16)
        n281 = call <vilib>:"NT Write Number.vi"("Numeric"=w434, "Name"=w433) -> ()  [unwired: 9 in, 1 out]
      }
      event "Test Ring": Value Change {
        # "When a test mode helper value is selected from the ring,\nset the tree item's variable to the string value"
        n282 = event-data() -> ("NewVal"=w443:u16)  [unwired: 1 in]
        n283 = property on="Test Ring" class="Ring (strict)"() -> ("Strings []"=w444:string[])  [unwired: 2 in, 2 out]
        n284 = Index Array(array=w444, index=w443) -> (element=w442:string)
        n285 = call <vilib>:"NT Write String.vi"("String"=w442, "Name"=w441) -> ()  [unwired: 9 in, 1 out]
      }
      event "Rec Mode": Value Change {
        # "Update globals for recording mode and path to read log from.\nClear when logging and let NetworkTables set path for vision to\nuse."
        n286 = event-data() -> ("NewVal"=w455:enum32{"Stop", "Record", "Playback"})  [unwired: 1 in]
        n287 = global write "WPI_DashboardLogging Global.vi" "Logging Filename"(path "") -> ()
        n288 = global write "WPI_DashboardLogging Global.vi" "Recording"(w455) -> ()
        n289 = case shown="\"Playback\"" w455 {
          tunnel: w454 -> [_ w457 w466]
          tunnel: [_ _ w465] -> w452
          tunnel: [_ _ w464] -> _
          tunnel: w450 -> [_ _ w462]
          tunnel: cluster{i32, i32} {-250, 170} -> [_ _ w461]
          tunnel: [_ _ T29 {"Image Size"=TRUE, "Image Type"=TRUE, "Pixel Value"=TRUE, "ROI Information"=TRUE, "Zoom Factor"=FALSE} ("Image Information Shown:All Elements")] -> w445
          tunnel: [_ _ TRUE ("Zoom Factor")] -> w446
          tunnel: w448 -> [_ _ w458]
          frame Default {
          }
          frame "Stop", "Record" {
            # "Place Window too"
            n290 = invoke class="VI" method="FP.Close"(reference=w457) -> (reference out=w456:refnum<vi>)  [unwired: 2 in, 2 out]
            n291 = invoke class="VI" method="Abort VI"(reference=w456) -> ()  [unwired: 2 in, 3 out]
          }
          frame "Playback" {
            n292 = call "Open Playback Panel.vi"("Offset"=w461, "DB VI Ref"=w462, "Playback in"=w466) -> ("Playback out"=w463:refnum<vi>)  [unwired: 8 in]
            n293 = register-events(w463, w458) -> (reference out=w465:refnum<event-registration>, error out=w464:errorcluster)  [unwired: 2 in]
          }
        }
        n294 = property on="Camera Image Right" class="ImageControl"("Image Information Shown"=w445, "Image Information Visible"=w446) -> ()  [unwired: 2 in, 2 out]
        n295 = property on="Camera Image" class="ImageControl"("Image Information Shown"=w445, "Image Information Visible"=w446) -> ()  [unwired: 2 in, 2 out]
        n296 = call <vilib>:"WPI_DashboardNT Log FieldName Cache.vi"("Operation"=enum16{"Lookup/Add", "Index", "Clear"}."Clear") -> ()  [unwired: 8 in, 3 out]
      }
      event Panel Close {
        w468 = enum32{"Stop", "Record", "Playback"}."Stop" ("Rec Mode")
        # "Playback window has been closed, abort"
        n297 = event-data() -> ()  [unwired: 1 in, 4 out]
        n298 = local write "Rec Mode"(w468) -> ()
        n299 = global write "WPI_DashboardLogging Global.vi" "Recording"(w468) -> ()
      }
      event Panel Close {
        # "Abort playback window and ourself"
        n300 = event-data() -> ()  [unwired: 1 in, 4 out]
        n301 = invoke class="VI" method="FP.Close"(reference=w472) -> (reference out=w471:refnum<vi>)  [unwired: 2 in, 2 out]
        n302 = invoke class="VI" method="Abort VI"(reference=w471) -> (error out=w470:errorcluster)  [unwired: 2 in, 2 out]
        n303 = invoke class="VI" method="Abort VI"(error in=w470) -> ()  [unwired: 2 in, 3 out]
      }
      event User Event {
        n304 = event-data() -> ("IDs"=w479:cluster{"RPC field ID":u16, "Unique ID":u16}, "String"=w478:string)  [unwired: 1 in]
        n305 = Bundle("IDs"=w479, "String"=w478) -> (w477:T9)  [unwired: 1 in]
        n306 = call <vilib>:"Retrieve RPC Response.vi"("RPC Response"=w477) -> ("Output"=w475:string[][])  [unwired: 10 in]
        n307 = Build Array (concatenate)(w473, w475) -> (w474:string[][])
        n308 = local write "Command Params"(w474) -> ()
        n309 = local write "Cmd Status"("" ("Cmd Status")) -> ()
      }
      event "Tree": Double Click {
        n310 = event-data() -> ("PlatMods"=w485:T32, "Tag"=w482:string)  [unwired: 1 in]
        n311 = Unbundle(w485) -> ("Shift"=w484:bool)  [unwired: 4 out]
        n312 = String Subset(string=w482, length (rest)=1 ("length (rest)")) -> (substring=w481:string)  [unwired: 1 in]
        n313 = Not(x=w484) -> (.not. x?=w483:bool)
        n314 = case shown="\"/\"" w481 {
          tunnel: w482 -> [_ w488]
          tunnel: w483 -> [_ w487]
          frame Default {
          }
          frame "/" {
            n315 = call <vilib>:"NT Update Persistence.vi"("Persistence"=w487, "Name"=w488) -> ()  [unwired: 9 in, 1 out]
          }
        }
      }
    }
  }
  n316 = while {
    tunnel: w70 -> [w490]
    i -> [w493]
    stop <- FALSE stop-if-true
    n317 = Wait (ms)(milliseconds to wait=u32 100) -> ()  [unwired: 1 out]
    n318 = case shown="\"Playback\"" "Rec Mode" {
      tunnel: w493 -> [_ _ w508]
      tunnel: [u32 2829099 ("Base Color") u32 11141120 ("Target Color") w497] -> w489
      frame "Stop", Default {
        # "Reset the color, extra updates don't cost much"
      }
      frame "Record" {
      }
      frame "Playback" {
        # "Playback"
        n319 = Quotient & Remainder(x=w508, y=u32 50 ("milliseconds to wait")) -> (x-y*floor(x/y)=w504:u32)  [unwired: 1 out]
        n320 = Divide(x=w504, y=u32 50 ("milliseconds to wait")) -> (x/y=w501:dbl)
        n321 = Multiply(x=6.283185307179586, y=w501) -> (x*y=w506:dbl)
        n322 = Sine(x=w506) -> (sin(x)=w505:dbl)
        n323 = Absolute Value(x=w505) -> (abs(x)=w498:dbl)
        n324 = call "Interpolate RGB Color.vi"("Proportion"=w498, "Target Color"=u32 30976, "Base Color"=u32 2829099) -> ("Result Color"=w497:u32)  [unwired: 8 in]
      }
    }
    n325 = property class="Pane"(reference=w490, "PaneColor"=w489) -> ()  [unwired: 1 in, 2 out]
  }
  n326 = local write "Dashboard Tab"(T2."Drive" ("Dashboard Tab")) -> ()
  n327 = property on="On/Off" class="Bool (strict)"("Visible"=w41) -> ()  [unwired: 2 in, 2 out]
  n328 = property on="Motor" class="Clust (strict)"("Visible"=w41) -> ()  [unwired: 2 in, 2 out]
  n329 = property on="Progress" class="Clust (strict)"("Visible"=w41) -> ()  [unwired: 2 in, 2 out]
  n330 = property on="Test Ring" class="Ring (strict)"("Visible"=w41) -> ()  [unwired: 2 in, 2 out]
  n331 = property on="Rev/Fwd" class="Clust (strict)"("Visible"=w41) -> ()  [unwired: 2 in, 2 out]
  n332 = while {
    tunnel: u16 1741 ("timeout ms (25000)") -> [w510]
    stop <- FALSE stop-if-true
    n333 = TCP Create Listener(10:w510) -> (0:w509:errorcluster, 3:w511:refnum<k5>)  [unwired: 4 in, 1 out]
    n334 = case shown="No Error" w509 {
      selector: w509 -> [w513 _]
      tunnel: w511 -> [w514 _]
      frame No Error {
        n335 = while {
          tunnel: w514 -> [w517]
          tunnel: w513 -> [w516]
          stop <- FALSE stop-if-true
          n336 = TCP Wait On Listener(8:w516, 11:w517) -> (0:w518:errorcluster, 4:w519:refnum<k5>)  [unwired: 2 in, 3 out]
          n337 = local write "TCP"(w519) -> ()
          n338 = case shown="No Error" w518 {
            frame No Error {
            }
            frame Error {
              n339 = Wait (ms)(milliseconds to wait=u32 1000) -> ()  [unwired: 1 out]
            }
          }
        }
      }
      frame Error {
        n340 = Wait (ms)(milliseconds to wait=u32 1000) -> ()  [unwired: 1 out]
      }
    }
  }
  n341 = local write "Command Selection"(u16 0 ("milliseconds to wait")) -> ()
  n342 = call <vilib>:"Close.vi"("Error In"=w2, "LINX Resource"=w1) -> ()  [unwired: 9 in, 1 out]
  n343 = local write "Command Params"(string[][] [] ("Command Params")) -> ()
  n344 = global write "WPI_DashboardLogging Global.vi" "Recording"(w64) -> ()
  n345 = local write "Rec Mode"(w64) -> ()
  n346 = call <vilib>:"NT Write String.vi"("String"="Select Auto", "Name"="Auto Selector") -> ()  [unwired: 9 in, 1 out]
